vi "Matches.vi"(8 "error in (no error)":errorcluster, 10 "Actual":variant, 11 "Error in":refnum<class "Error.lvclass">) -> (0 "error out":errorcluster, 2 "Result":bool, 3 "Error out":refnum<class "Error.lvclass">)   [LabVIEW 2017, in "Transparent Assertions.lvlib" / "Constraints.lvlib" / "Error.lvclass"]
doc: "Evaluates the constraint for <B>Actual</B>. Returns true if the constraint is met."
uses:
  Error.lvclass
  ErrorType.ctl
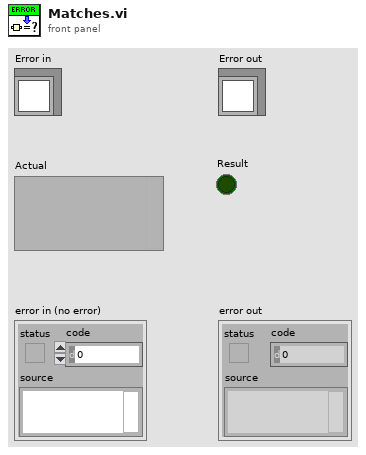
[diagram p1: front panel]
types:
  T1 = typedef "Transparent Assertions.lvlib/Constraints.lvlib/Error.lvclass/ErrorType.ctl" = enum16{"error", "warning", "no error"}
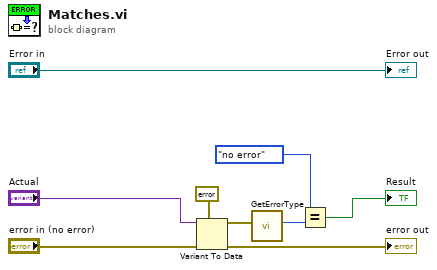
[diagram p0: block diagram]
diagram:
  n1 = Variant To Data(error in="error in (no error)", type=errorcluster {"status"=FALSE, "code"=0, "source"=""} ("error constant"), Variant="Actual") -> (data=w5:errorcluster, error out=→"error out":errorcluster)
  n2 = call "GetErrorType.vi"("error in (no error)"=w5) -> ("ErrorType"=w2:T1)  [unwired: 10 in]
  n3 = Equal?(x=ErrorType."no error", y=w2) -> (x = y?=→"Result":bool)
  "Error out" <- "Error in"
